vi "Movement Sequence.vi"(8 "AI5 Setpoint":dbl, 9 "PWM 7 In":dbl, 10 "PWM 5 In":dbl, 11 "Moving Up? (setpoint)":bool) -> (0 "PWM 5 Out":dbl, 2 "PWM 7 Out":dbl)   [LabVIEW 2011]
uses:
  Robot Global Data.vi
panel:
  in  "Rotation Sequence":dbl
  in  "Move Down State Control":dbl
  in  "Move Up State Control":dbl
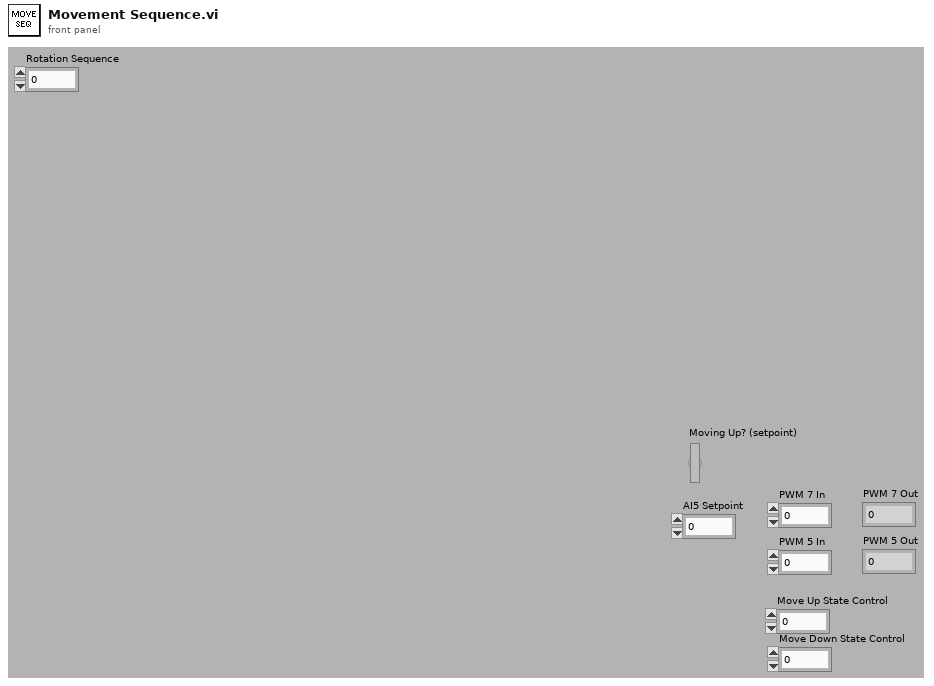
[diagram p1: front panel]
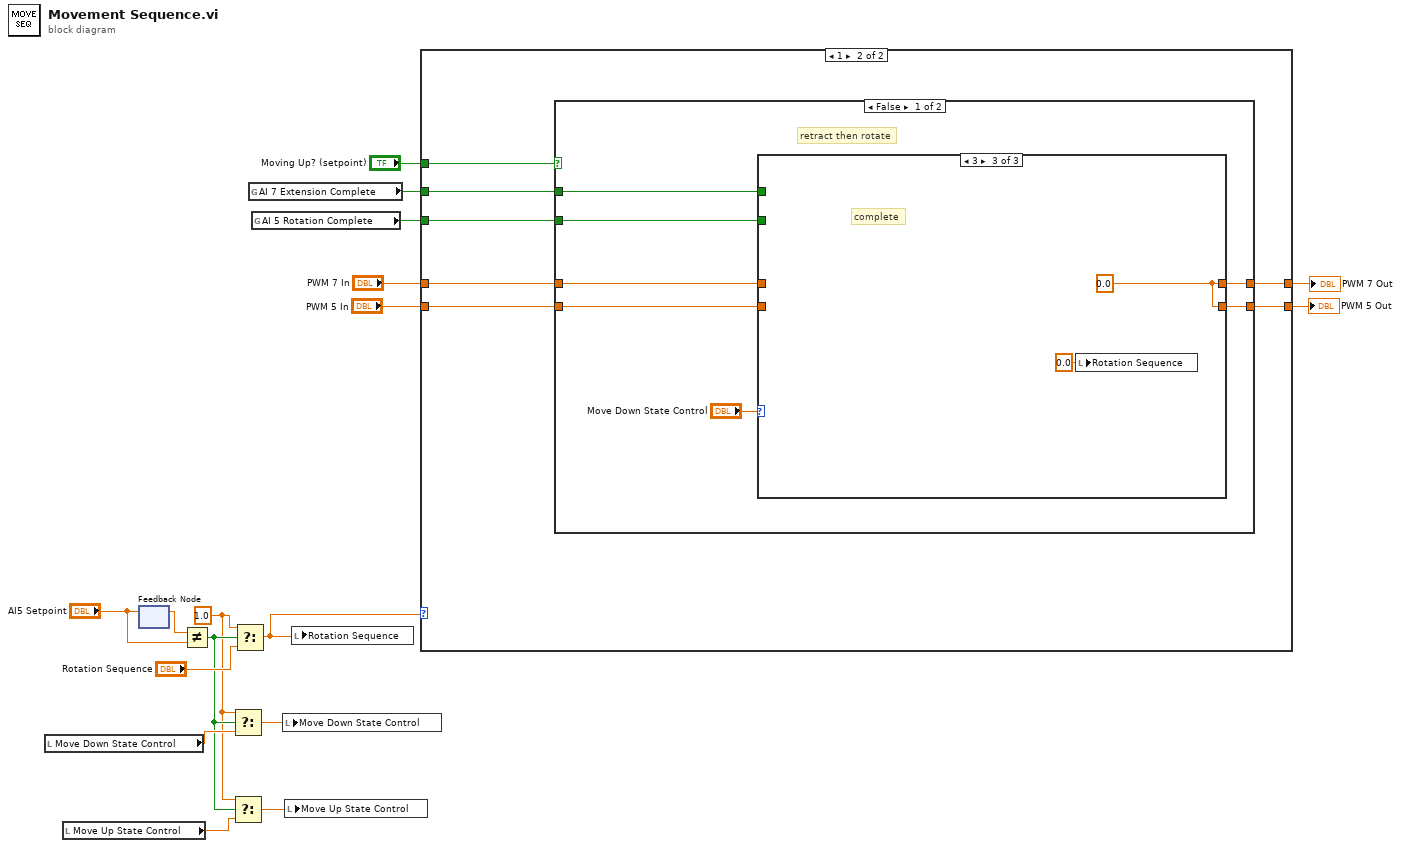
[diagram p0: block diagram]
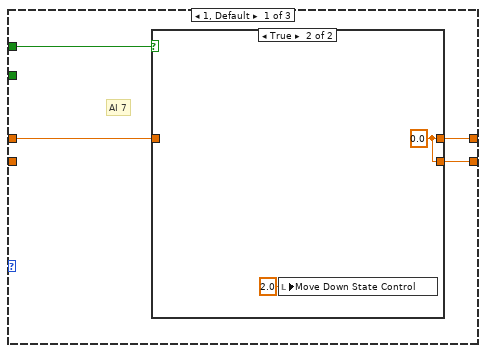
[diagram p3: hidden frame]
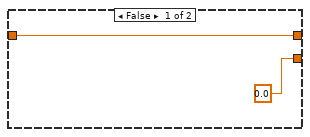
[diagram p4: hidden frame]
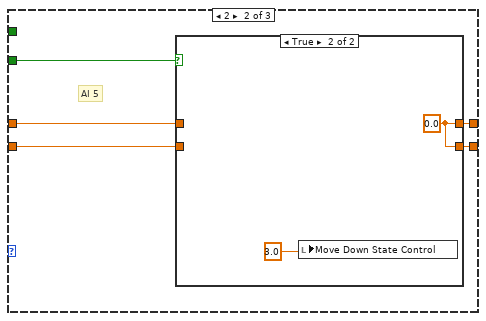
[diagram p5: hidden frame]
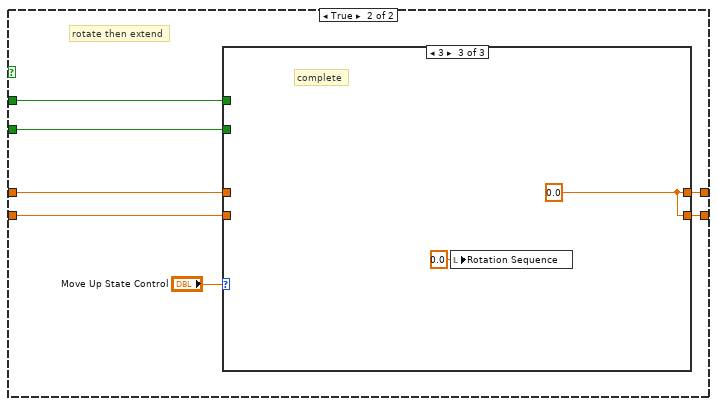
[diagram p7: hidden frame]
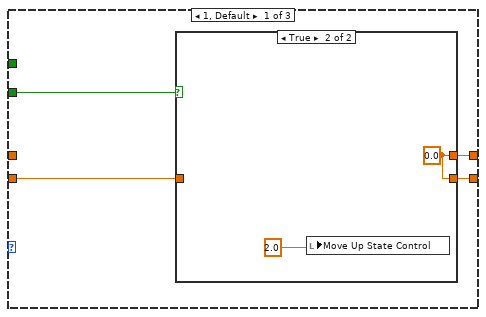
[diagram p8: hidden frame]
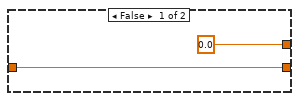
[diagram p9: hidden frame]
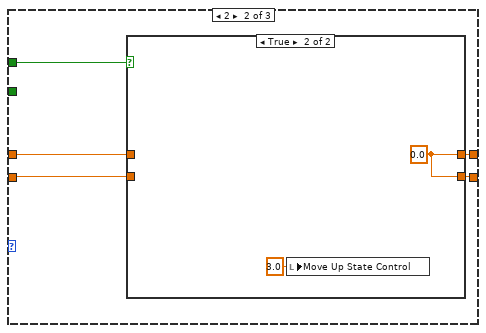
[diagram p10: hidden frame]
diagram:
  w5 = 1.0 ("t")
  n1 = local read "Move Down State Control"() -> (w7:dbl)
  n2 = local read "Move Up State Control"() -> (w4:dbl)
  n3 = feedback-in #1("AI5 Setpoint") -> ()
  n4 = feedback #1() -> (w1:dbl)  [unwired: 1 out]
  n5 = Not Equal?(x=w1, y="AI5 Setpoint") -> (x != y?=w6:bool)
  n6 = Select(t=w5, s=w6, f=w7) -> (s? t:f=w8:dbl)
  n7 = Select(t=w5, s=w6, f=w4) -> (s? t:f=w3:dbl)
  n8 = Select(t=w5, s=w6, f="Rotation Sequence") -> (s? t:f=w9:dbl)
  n9 = global read "Robot Global Data.vi" "AI 7 Extension Complete"() -> (w13:bool)
  n10 = global read "Robot Global Data.vi" "AI 5 Rotation Complete"() -> (w12:bool)
  n11 = local write "Move Down State Control"(w8) -> ()
  n12 = local write "Move Up State Control"(w3) -> ()
  n13 = local write "Rotation Sequence"(w9) -> ()
  n14 = case shown="1" w9 {
    tunnel: "PWM 5 In" -> [w18 w26]
    tunnel: [w18 w25] -> w16
    tunnel: [w19 w24] -> w15
    tunnel: "PWM 7 In" -> [w19 w23]
    tunnel: w13 -> [_ w22]
    tunnel: w12 -> [_ w21]
    tunnel: "Moving Up? (setpoint)" -> [_ w20]
    frame 0, Default {
    }
    frame 1 {
      n15 = case shown="False" w20 {
        tunnel: w26 -> [w31 w59]
        tunnel: [w29 w58] -> w25
        tunnel: [w30 w57] -> w24
        tunnel: w23 -> [w32 w55]
        tunnel: w22 -> [w28 w54]
        tunnel: w21 -> [w27 w53]
        frame False {
          # "retract then rotate"
          n16 = case shown="3" "Move Down State Control" {
            tunnel: w31 -> [_ w46 _]
            tunnel: [w37 w45 w52] -> w29
            tunnel: [w36 w44 w52] -> w30
            tunnel: w32 -> [w35 w43 _]
            tunnel: w28 -> [w34 _ _]
            tunnel: w27 -> [_ w42 _]
            frame 1, Default {
              # "AI 7"
              n17 = case shown="True" w34 {
                tunnel: [0.0 ("Rotation In") w40] -> w37
                tunnel: [w38 w40] -> w36
                tunnel: w35 -> [w38 _]
                frame False {
                }
                frame True {
                  w40 = 0.0 ("Extension In")
                  n18 = local write "Move Down State Control"(2.0 ("Move Up State Control")) -> ()
                }
              }
            }
            frame 2 {
              # "AI 5"
              n19 = case shown="True" w42 {
                tunnel: w46 -> [w48 _]
                tunnel: [w48 w49] -> w45
                tunnel: [w47 w49] -> w44
                tunnel: w43 -> [w47 _]
                frame False {
                }
                frame True {
                  w49 = 0.0
                  n20 = local write "Move Down State Control"(3.0 ("Move Up State Control")) -> ()
                }
              }
            }
            frame 3 {
              w52 = 0.0 ("Extension In")
              # "complete"
              n21 = local write "Rotation Sequence"(0.0 ("Rotation Sequence")) -> ()
            }
          }
        }
        frame True {
          # "rotate then extend"
          n22 = case shown="3" "Move Up State Control" {
            tunnel: w59 -> [w63 w69 _]
            tunnel: [w62 w72 w78] -> w58
            tunnel: [w61 w71 w78] -> w57
            tunnel: w55 -> [_ w70 _]
            tunnel: w54 -> [_ w68 _]
            tunnel: w53 -> [w60 _ _]
            frame 1, Default {
              n23 = case shown="True" w60 {
                tunnel: w63 -> [w64 _]
                tunnel: [w64 w66] -> w62
                tunnel: [0.0 w66] -> w61
                frame False {
                }
                frame True {
                  w66 = 0.0
                  n24 = local write "Move Up State Control"(2.0 ("Move Up State Control")) -> ()
                }
              }
            }
            frame 2 {
              n25 = case shown="True" w68 {
                tunnel: [w73 w75] -> w72
                tunnel: [w74 w75] -> w71
                tunnel: w70 -> [w74 _]
                tunnel: w69 -> [w73 _]
                frame False {
                }
                frame True {
                  w75 = 0.0 ("Rotation In")
                  n26 = local write "Move Up State Control"(3.0 ("Move Up State Control")) -> ()
                }
              }
            }
            frame 3 {
              w78 = 0.0 ("Extension In")
              # "complete"
              n27 = local write "Rotation Sequence"(0.0 ("Rotation Sequence")) -> ()
            }
          }
        }
      }
    }
  }
  "PWM 5 Out" <- w16
  "PWM 7 Out" <- w15
